vi "Pract_1.vi"() -> ()   [LabVIEW 2022 SP3]
panel:
  in  "Número A":dbl
  in  "Número B":dbl
  in  "?":T1(tab)
  out "Suma":dbl
  out "Positiva":bool
  out "Negativa":bool
  out "Resta":dbl
  out "Negativa":bool
  out "Positiva":bool
  out "Multiplicación":dbl
  out "?":dbl(knob) scale=0.0..1000.0
  out "Por debajo":dbl
  out "Por encima":dbl
  out "Más cercano":dbl
  out "División":dbl
  out "RESIDUO":u8(slide) scale=0.0..50.0
  out "COCIENTE":dbl(slide) scale=0.0..100.0
  # "NÚMEROS A OPERAR"
  # "REDONDEO"
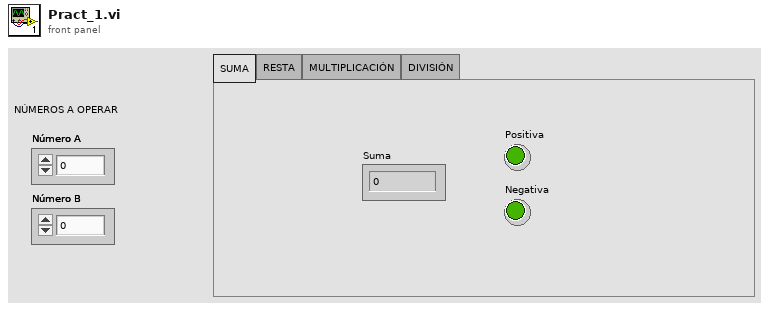
[diagram p1: front panel]
types:
  T1 = enum32{"SUMA", "RESTA", "MULTIPLICACIÓN", "DIVISIÓN"}
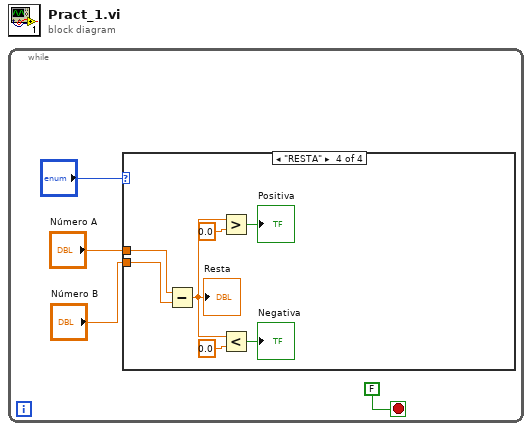
[diagram p0: block diagram]
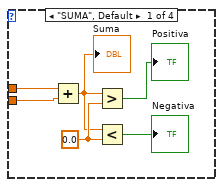
[diagram p2: hidden frame]
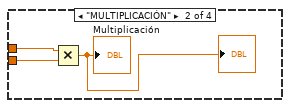
[diagram p3: hidden frame]
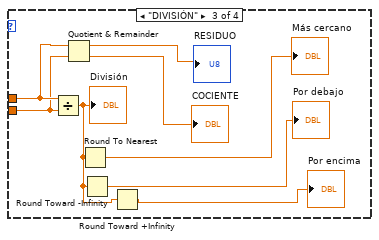
[diagram p4: hidden frame]
diagram:
  n1 = while {
    stop <- FALSE stop-if-true
    n2 = case shown="\"RESTA\"" "?" {
      tunnel: "Número A" -> [w10 w13 w21 w28]
      tunnel: "Número B" -> [w9 w12 w20 w27]
      frame "SUMA", Default {
        w8 = 0.0 ("y")
        n3 = Add(x=w10, y=w9) -> (x+y=w7:dbl)
        "Suma" <- w7
        n4 = Greater?(x=w7, y=w8) -> (0:→"Positiva":bool)
        n5 = Less?(x=w7, y=w8) -> (x < y?=→"Negativa":bool)
      }
      frame "MULTIPLICACIÓN" {
        n6 = Multiply(x=w13, y=w12) -> (x*y=→"Multiplicación" →"?":dbl)
      }
      frame "DIVISIÓN" {
        n7 = Divide(x=w21, y=w20) -> (x/y=w15:dbl)
        "División" <- w15
        n8 = Quotient & Remainder(x=w21, y=w20) -> (x-y*floor(x/y)=→"RESIDUO":dbl, floor(x/y)=→"COCIENTE":dbl)
        n9 = Round To Nearest(number=w15) -> (nearest integer value=→"Más cercano":dbl)
        n10 = Round Toward -Infinity(1:w15) -> (0:→"Por debajo":dbl)
        n11 = Round Toward +Infinity(x=w15) -> (ceil(x): smallest int >= x=→"Por encima":dbl)
      }
      frame "RESTA" {
        n12 = Subtract(x=w28, y=w27) -> (x-y=w24:dbl)
        "Resta" <- w24
        n13 = Greater?(x=w24, y=0.0) -> (0:→"Positiva":bool)
        n14 = Less?(x=w24, y=0.0) -> (x < y?=→"Negativa":bool)
      }
    }
  }
